vi "Write Packet.vi"(8 "error in (no error)":errorcluster, 9 "SessionMailbox in":refnum<queue>, 10 "Outgoing":T1, 11 "MQTT_Base in":refnum<class "MQTT_Base.lvclass">) -> (0 "error out":errorcluster, 3 "MQTT_Base out":refnum<class "MQTT_Base.lvclass">)   [LabVIEW 2013, in "MQTT Server.lvlib" / "MQTT_Base.lvclass"]
uses:
  MQTT_Base/MQTT_Base.lvclass
  MQTT_Base/Response -- cluster.ctl
  Control Packets/ControlPacket/ControlPacket.lvclass
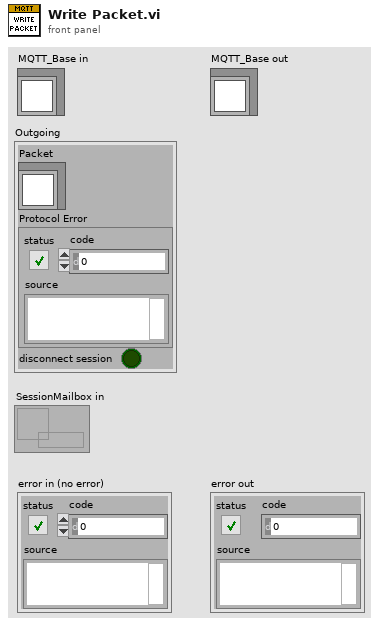
[diagram p1: front panel]
types:
  T1 = typedef "MQTT Server.lvlib/MQTT_Base.lvclass/Response -- cluster.ctl" = cluster{"Packet":refnum<class "ControlPacket.lvclass">, "Protocol Error":errorcluster, "disconnect session":bool}
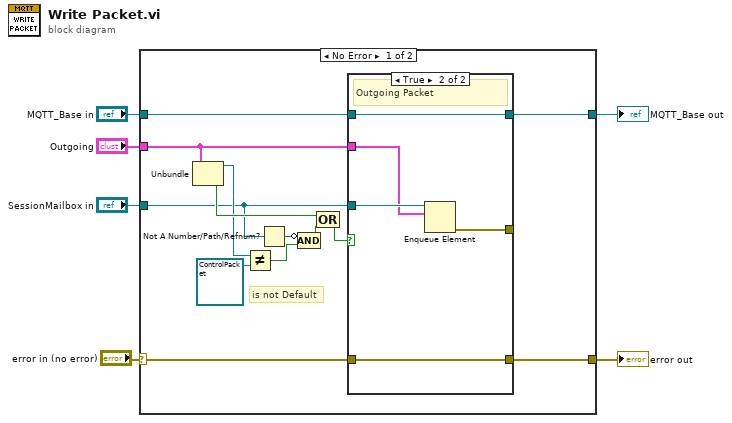
[diagram p0: block diagram]
diagram:
  n1 = case shown="No Error" "error in (no error)" {
    selector: "error in (no error)" -> [w7 w28]
    tunnel: "Outgoing" -> [w15 _]
    tunnel: "SessionMailbox in" -> [w14 _]
    tunnel: [w13 w28] -> w4
    tunnel: [w12 w27] -> w3
    tunnel: "MQTT_Base in" -> [w11 w27]
    frame No Error {
      # "is not Default"
      n2 = Unbundle(w15) -> ("Packet"=w16:refnum<class "ControlPacket.lvclass">, "disconnect session"=w17:bool)  [unwired: 1 out]
      n3 = Not Equal?(x=w16, y=refnum<class "ControlPacket.lvclass"> refnum ("ControlPacket.lvclass")) -> (x != y?=w10:bool)
      n4 = Not A Number/Path/Refnum?(number/path/refnum=w14) -> (NaN/Path/Refnum?=w9:bool)
      n5 = Compound Arithmetic op=AND(invert w9, w10) -> (w18:bool)
      n6 = Compound Arithmetic op=OR(w17, w18) -> (w19:bool)
      n7 = case shown="True" w19 {
        tunnel: w15 -> [_ w22]
        tunnel: w14 -> [_ w26]
        tunnel: w7 -> [w20 w24]
        tunnel: w11 -> [w21 w25]
        tunnel: [w21 w25] -> w12
        tunnel: [w20 w24] -> w13
        tunnel: [_ w23] -> _
        frame False {
        }
        frame True {
          # "Outgoing Packet"
          n8 = Enqueue Element(queue=w26, element=w22) -> (error out=w23:errorcluster)  [unwired: 2 in, 2 out]
        }
      }
    }
    frame Error {
      # "#Question: \nOn Server Error, should we try to close all sessions here\nor let the destroy method do that."
    }
  }
  "error out" <- w4
  "MQTT_Base out" <- w3
